vi "OP300ZP_CONTI.vi"(0 "VISA":refnum<visa-resource-name>, 3 "ERRIN":errorcluster caption="entrée d'erreur (pas d'erreur)") -> (7 "DATA OUT":string, 8 "Conti (mOhms)":dbl format="%#_10f", 9 "Conti (Ohms)":dbl format="%#_10f", 10 "ERROUT2":errorcluster caption="sortie d'erreur")   [LabVIEW 2020]
uses:
  R_VG.vi
  <vilib>/Instr/_visa.llb/VISA Configure Serial Port (Instr).vi
panel:
  out "nombre renvoyé 2":u32
  out "ERROUT":errorcluster caption="sortie d'erreur"
  out "ERR_ADJ":string="La mise à zéo n'a pas été effectuée"
  in  "Arrêter":bool
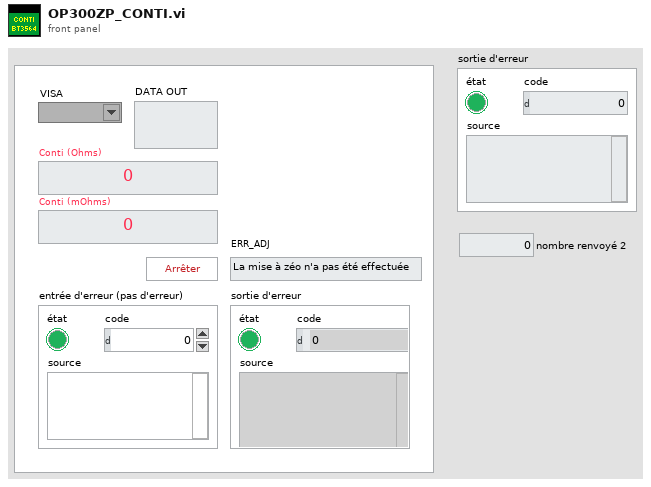
[diagram p1: front panel]
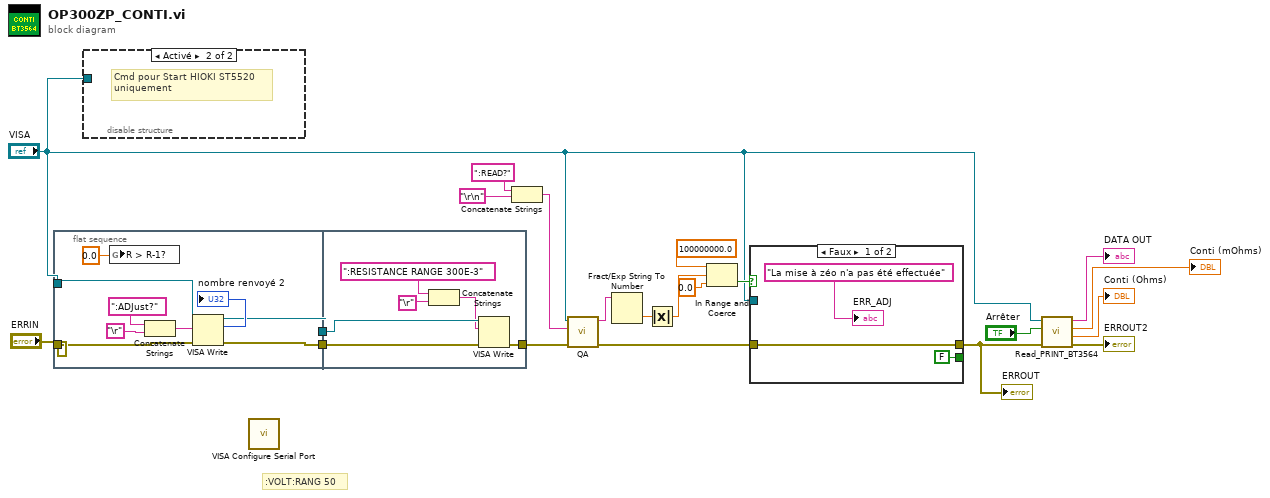
[diagram p0: block diagram]
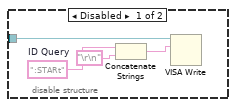
[diagram p2: hidden frame]
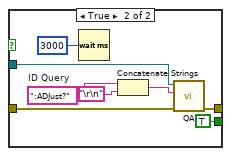
[diagram p3: hidden frame]
diagram:
  # ":VOLT:RANG 50"
  n1 = flat-sequence {
    tunnel: "ERRIN" -> [w29]
    tunnel: "VISA" -> [w28]
    tunnel: [w25] -> w2
    tunnel: [w26] -> w1
    tunnel: [w35] -> w7
    tunnel: w2 -> [w35]
    tunnel: w1 -> [w34]
    frame #0 {
      n2 = global write "R_VG.vi" "R > R-1?"(0.0 ("R > R-1?")) -> ()
      n3 = Concatenate Strings(":ADJust?" ("Command"), "\r") -> (w22:string)
      n4 = VISA Write(VISA resource name=w28, write buffer=w22, error in (no error)=w29) -> (VISA resource name out=w26:refnum<visa-resource-name>, return count=→"nombre renvoyé 2":u32, error out=w25:errorcluster)
    }
    frame #1 {
      n5 = Concatenate Strings(":RESISTANCE RANGE 300E-3" ("chaîne"), "\r") -> (w31:string)
      n6 = VISA Write(VISA resource name=w34, write buffer=w31) -> ()  [unwired: 1 in, 3 out]
    }
  }
  n7 = disable-structure shown="Activé" {
    disable-tunnel: "VISA" -> [w39 _]
    frame Disabled {
      w37 = ":STARt"  # ID Query
      n8 = Concatenate Strings(w37, "\r\n") -> (w38:string)
      n9 = VISA Write(VISA resource name=w39, write buffer=w38) -> ()  [unwired: 1 in, 3 out]
    }
    frame Enabled {
      # "Cmd pour Start HIOKI ST5520 \nuniquement"
    }
  }
  n10 = call-poly "VISA Configure Serial Port"() -> ()  [unwired: 14 in, 2 out]
  n11 = Concatenate Strings(":READ?" ("ID Query"), "\r\n") -> (w20:string)
  n12 = call "QA.vi"("ERRIN"=w7, "Chaîne"=w20, "VISA"="VISA") -> ("ERROUT"=w16:errorcluster, "DATA OUT"=w5:string)  [unwired: 7 in]
  n13 = Fract/Exp String To Number(string=w5) -> (number=w14:dbl)  [unwired: 3 in, 1 out]
  n14 = Absolute Value(x=w14) -> (abs(x)=w13:dbl)
  n15 = In Range and Coerce(upper limit=100000000.0 ("limite supérieure"), x=w13, lower limit=0.0 ("limite inférieure")) -> (In Range?=w17:bool)  [unwired: 1 out]
  n16 = case shown="Faux" w17 {
    tunnel: w16 -> [w42 w48]
    tunnel: [w42 w47] -> w15
    tunnel: "VISA" -> [_ w45]
    tunnel: [FALSE TRUE] -> _
    frame False {
      "ERR_ADJ" <- "La mise à zéo n'a pas été effectuée"
    }
    frame True {
      w49 = ":ADJust?"  # ID Query
      n17 = Wait (ms)(milliseconds to wait=u32 3000 ("attente (ms)")) -> ()  [unwired: 1 out]
      n18 = Concatenate Strings(w49, "\r\n") -> (w46:string)
      n19 = call "QA.vi"("ERRIN"=w48, "Chaîne"=w46, "VISA"=w45) -> ("ERROUT"=w47:errorcluster)  [unwired: 7 in, 1 out]
    }
  }
  "ERROUT" <- w15
  n20 = call "Read_PRINT_BT3564.vi"("ERRIN"=w15, "Arrêter"="Arrêter", "VISA"="VISA") -> ("errout"=→"ERROUT2":errorcluster, "Conti (Ohms)"=→"Conti (Ohms)":dbl, "Conti (mOhms)"=→"Conti (mOhms)":dbl, "DATA OUT"=→"DATA OUT":string)  [unwired: 5 in]
